vi "HFRR ADV v05.vi"() -> ()   [LabVIEW 2025] (continued)
    n981 = local read "Re-Initialise"() -> (w1097:bool)
    n982 = local read "Main Tab"() -> (w1093:T2)
    n983 = local read "service 3"() -> (w1094:bool)
    n984 = local read "OPEN 6"() -> (w1096:bool)
    n985 = local read "EDIT 2"() -> (w1099:bool)
    n986 = local read "RUN"() -> (w1111:bool)
    n987 = local read "RUN"() -> (w1109:bool)
    n988 = disable-structure shown="Disabled" {
      disable-tunnel: [w1126 _] -> w1091
      disable-tunnel: [w1125 _] -> w1089
      frame Disabled {
        n989 = local read "Temperature before test"() -> (w1119:dbl)
        n990 = local read "Temperature after test"() -> (w1132:dbl)
        n991 = case shown="True" "Save Results" {
          frame False {
          }
          frame True {
            w1148 = "\r"
            n992 = local write "Save Results"(FALSE ("OK Button 5")) -> ()
            n993 = local read "Temperature before test"() -> (w1186:dbl)
            n994 = local read "Temperature after test"() -> (w1188:dbl)
            n995 = local read "Humidity before test"() -> (w1185:dbl)
            n996 = local read "Humidity after test"() -> (w1187:dbl)
            n997 = local read "WS1.4"() -> (w1192:dbl)
            n998 = local read "AVP"() -> (w1190:dbl)
            n999 = Number To Fractional String(number=w1192, width (-)=i16 6, precision (6)=i16 1) -> (F-format string=w1152:string)  [unwired: 1 in]
            n1000 = local read "MWSD"() -> (w1189:dbl)
            n1001 = local read "String"() -> (w1181:string)
            n1002 = local read "FILE"() -> (w1184:string)
            n1003 = local read "HCF"() -> (w1191:dbl)
            n1004 = Number To Fractional String(number=w1185, width (-)=i16 6, precision (6)=i16 1) -> (F-format string=w1177:string)  [unwired: 1 in]
            n1005 = Number To Fractional String(number=w1186, width (-)=i16 6, precision (6)=i16 1) -> (F-format string=w1174:string)  [unwired: 1 in]
            n1006 = Number To Fractional String(number=w1187, width (-)=i16 6, precision (6)=i16 1) -> (F-format string=w1170:string)  [unwired: 1 in]
            n1007 = Number To Fractional String(number=w1188, width (-)=i16 6, precision (6)=i16 1) -> (F-format string=w1166:string)  [unwired: 1 in]
            n1008 = Number To Fractional String(number=w1190, width (-)=i16 6, precision (6)=i16 3) -> (F-format string=w1159:string)  [unwired: 1 in]
            n1009 = Concatenate Strings(w1181, w1184) -> (w1203:string)
            n1010 = Number To Fractional String(number=w1189, width (-)=i16 6, precision (6)=i16 1) -> (F-format string=w1163:string)  [unwired: 1 in]
            n1011 = Number To Fractional String(number=w1191, width (-)=i16 6, precision (6)=i16 2) -> (F-format string=w1157:string)  [unwired: 1 in]
            n1012 = Concatenate Strings("(" ("string"), w1152, ")Microns" ("string")) -> (w1151:string)
            n1013 = local read "REMARKS"() -> (w1183:string)
            "REMARKS 2" <- w1183
            n1014 = Concatenate Strings("(" ("string"), w1177, " ) % RH," ("string")) -> (w1178:string)
            n1015 = Concatenate Strings(w1157, ")" ("string")) -> (w1155:string)
            n1016 = Concatenate Strings("(" ("string"), w1174, ")  Deg C ," ("string")) -> (w1173:string)
            n1017 = Concatenate Strings("(" ("string"), w1170, " ) % RH," ("string")) -> (w1169:string)
            n1018 = Concatenate Strings("(" ("string"), w1166, ")  Deg C ," ("string")) -> (w1165:string)
            n1019 = Concatenate Strings("(" ("string"), w1163, ")  Microns," ("string")) -> (w1162:string)
            n1020 = Concatenate Strings("(" ("string"), w1159, ")  kPa," ("string")) -> (w1149:string)
            n1021 = Concatenate Strings(w1203, ".dwm" ("Substring")) -> (w1201:string)
            n1022 = String To Path(string=w1201) -> (path=w1200:path)
            n1023 = Concatenate Strings(w1183, w1148, " Humidity before test= " ("Substring"), w1178, w1148, " Temperature before test = " ("Substring"), w1173, w1148, " Humidity after test= " ("Substring"), w1169, w1148, "Temperature after test = " ("Substring"), w1165, w1148, "MSD = " ("Substring"), w1162, w1148, "  AVP = " ("Substring"), w1149, w1148, "  HCF                     =( " ("Substring"), w1155, w1148, " WS1.4                  = " ("Substring"), w1151, w1148) -> (w1147:string)
            "data" <- w1147
            n1024 = call <vilib>:"Write Characters To File.vi"("append to file? (new file:F)"=FALSE, "character string"=w1147, "file path (dialog if empty)"=w1200) -> ()  [unwired: 2 in, 1 out]
            n1025 = Match Pattern(string=w1147, regular expression="!") -> (after substring=→"export":string)  [unwired: 1 in, 3 out]
          }
        }
        n1026 = Add(x=231.864, y=w1119) -> (x+y=w1116:dbl)
        n1027 = Add(x=231.864, y=w1132) -> (x+y=w1129:dbl)
        n1028 = Divide(x=1705.984, y=w1116) -> (x/y=w1117:dbl)
        n1029 = Divide(x=1705.984, y=w1129) -> (x/y=w1130:dbl)
        n1030 = local read "Humidity before test"() -> (w1121:dbl)
        n1031 = local read "Humidity after test"() -> (w1134:dbl)
        n1032 = Subtract(x=8.017352 ("y"), y=w1117) -> (x-y=w1143:dbl)
        n1033 = Subtract(x=8.017352 ("y"), y=w1130) -> (x-y=w1137:dbl)
        n1034 = expression code="10**y"(w1143) -> (w1123:dbl)
        n1035 = expression code="10**y"(w1137) -> (w1136:dbl)
        n1036 = Multiply(x=w1121, y=w1123) -> (x*y=w1122:dbl)
        n1037 = Multiply(x=w1134, y=w1136) -> (x*y=w1135:dbl)
        n1038 = Divide(x=w1122, y=750.0) -> (x/y=w1138:dbl)
        n1039 = Divide(x=w1135, y=750.0) -> (x/y=w1139:dbl)
        n1040 = Add(x=w1138, y=w1139) -> (x+y=w1140:dbl)
        n1041 = Divide(x=w1140, y=2.0) -> (x/y=w1142:dbl)
        n1042 = local write "AVP"(w1142) -> ()
        n1043 = Subtract(x=1.4, y=w1142) -> (x-y=w1125:dbl)
        n1044 = local read "HCF"() -> (w1126:dbl)
      }
      frame Enabled {
      }
    }
    n1045 = case shown="True" "EDIT 3" {
      frame False {
      }
      frame True {
        n1046 = local write "EDIT 3"(FALSE ("EDIT 3")) -> ()
        n1047 = local write "Main Tab"(T2."About" ("Main Tab")) -> ()
      }
    }
    n1048 = case shown="True" w1097 {
      frame False {
      }
      frame True {
        n1049 = local write "Re-Initialise"(FALSE ("Re-Initialise")) -> ()
      }
    }
    n1050 = case shown="False" w1111 {
      frame False {
        n1051 = local read "stopT"() -> (w2092:bool)
        n1052 = case shown="True" w2092 {
          frame False {
          }
          frame True {
            w2093 = FALSE
            n1053 = local write "stopT"(w2093) -> ()
            n1054 = local write "st enable"(w2093) -> ()
          }
        }
      }
      frame True {
        "stopT" <- TRUE
      }
    }
    n1055 = case shown="True" w1109 {
      frame False {
      }
      frame True {
        n1056 = local read "Main Tab"() -> (w2090:T2)
        n1057 = case shown="\"Compare Files\"" w2090 {
          frame "Acquire", Default {
          }
          frame "Compare Files" {
            n1058 = local write "Main Tab"(T2."Acquire" ("Main Tab")) -> ()
          }
          frame "About" {
          }
        }
      }
    }
    n1059 = case shown="True" w1099 {
      frame False {
        n1060 = property on="Password 2" class="Str"("Visible"=FALSE) -> ()  [unwired: 2 in, 2 out]
        n1061 = local write "Password 2"("" ("Password")) -> ()
      }
      frame True {
        n1062 = property on="Password 2" class="Str"("Visible"=TRUE) -> ()  [unwired: 2 in, 2 out]
        n1063 = Equal?(x="Password 2", y="HFRR1234") -> (x = y?=w1232:bool)
        n1064 = case shown="True" w1232 {
          tunnel: "Password 2" -> [w1235 _]
          frame False {
            n1065 = String Length(string=w1235) -> (length=w1236:i32)
            n1066 = Greater Than 0?(x=w1236) -> (x > 0?=w1234:bool)
            n1067 = case shown="False" w1234 {
              frame False {
                n1068 = property on="Password 2" class="Str"("Caption.Text"="Password (Advance Setting)") -> ()  [unwired: 2 in, 2 out]
              }
              frame True {
                n1069 = property on="Password 2" class="Str"("Caption.Text"="Incorrect Password!") -> ()  [unwired: 2 in, 2 out]
              }
            }
          }
          frame True {
            n1070 = local write "EDIT 2"(FALSE ("EDIT 2")) -> ()
            n1071 = local write "Password 2"("" ("Password")) -> ()
            n1072 = local write "Main Tab"(T2."Advance" ("Main Tab")) -> ()
          }
        }
      }
    }
    n1073 = case shown="True" "Prog Uno" {
      frame False {
      }
      frame True {
        n1074 = stacked-sequence {
          frame #0 {
            n1075 = Delete(path (use dialog)=path "C:/LAB-IQ-NXT/UNOCOMPILE.bat" ("working directory")) -> ()  [unwired: 4 in, 3 out]
          }
          frame #1 {
            n1076 = local read "Com Port 1"() -> (w1696:refnum<visa-resource-name>)
            n1077 = Concatenate Strings("cmd.exe /c \"mode " ("command line"), w1696, ":1200,n,8,1\"\n" ("command line")) -> (w1701:string)
            n1078 = Concatenate Strings(w1701, "CD\\\nCD WinDucom\navrdude -C avrdude.conf -v -patmega328p -carduino -P" ("command line"), w1696, " -b115200 -D -Uflash:w:UNO_V20.hex:i\n" ("command line"), "\r") -> (w1703:string)
            "STR" <- w1703
            n1079 = call <vilib>:"Write Characters To File.vi"("append to file? (new file:F)"=FALSE, "character string"=w1703, "file path (dialog if empty)"=path "C:/LAB-IQ-NXT/UNOCOMPILE.bat" ("working directory")) -> ()  [unwired: 2 in, 1 out]
          }
          frame #2 {
            n1080 = disable-structure shown="Disabled" {
              frame Disabled {
                w1707 = "cmd.exe  /c \"C:\\LAB-IQ-NXT\\UNOCOMPILE.bat\"" ("string")
                n1081 = local write "Prog Uno"(FALSE ("run minimized? (F)")) -> ()
                n1082 = call <vilib>:"System Exec.vi"("expected output size  (4096)"=u32 65535, "run minimized? (F)"=FALSE, "wait until completion? (T)"=TRUE ("run minimized? (F)"), "working directory"=path "C:/LAB-IQ-NXT", "standard input"=w1707, "command line"=w1707) -> ("error out"=w1706:errorcluster, "standard output"=→"String 42":string)  [unwired: 2 in, 2 out]
                "error out 3" <- w1706
                n1083 = flat-sequence {
                  tunnel: w1706 -> [_]
                  frame #0 {
                  }
                }
              }
              frame Enabled {
              }
            }
          }
        }
      }
    }
    n1084 = case shown="\"CEC F-096-A-06\"" "TEST STANDARD" {
      tunnel: [2.0 ("Set Temp") 0.0 ("Set Temp") 2.0 ("Set Temp") 0.0 ("Set Temp")] -> w1100
      frame "ASTM D6079", Default {
        # "astm hide"
        n1085 = local write "NORMAL LOAD"(2.0 ("NORMAL LOAD")) -> ()
        n1086 = local write "Set Strk"(1.0 ("Set Strk")) -> ()
        n1087 = local write "Set Hz"(50.0 ("Hz")) -> ()
        n1088 = local write "Set Temp"(60.0 ("Set Temp")) -> ()
        n1089 = local write "Set Rh"(53.0 ("Set Rh")) -> ()
        n1090 = local write "test time"(75.0 ("test time")) -> ()
        "Test Standard" <- "ASTM D6079" ("Test Standard 2")
      }
      frame "ISO 12156" {
        n1091 = local write "Set Strk"(1.0 ("Set Strk")) -> ()
        n1092 = local write "NORMAL LOAD"(2.0 ("NORMAL LOAD")) -> ()
        n1093 = local write "Set Temp"(60.0 ("Set Temp")) -> ()
        n1094 = local write "test time"(75.0 ("test time")) -> ()
        n1095 = local write "Set Hz"(50.0 ("Hz")) -> ()
        n1096 = local write "Set Rh"(53.0 ("Set Rh")) -> ()
      }
      frame "CEC F-096-A-06" {
        n1097 = local write "Set Strk"(1.0 ("Set Strk")) -> ()
        n1098 = local write "NORMAL LOAD"(2.0 ("NORMAL LOAD")) -> ()
        n1099 = local write "Set Temp"(60.0 ("Set Temp")) -> ()
        n1100 = local write "test time"(75.0 ("test time")) -> ()
        n1101 = local write "Set Hz"(50.0 ("Hz")) -> ()
        n1102 = local write "Set Rh"(53.0 ("Set Rh")) -> ()
      }
      frame "Custom" {
      }
    }
    n1103 = case shown="True" "Prog Due" {
      frame False {
      }
      frame True {
        n1104 = stacked-sequence {
          frame #0 {
            n1105 = Delete(path (use dialog)=path "C:/LAB-IQ-NXT/DUECOMPILE.bat" ("working directory")) -> ()  [unwired: 4 in, 3 out]
          }
          frame #1 {
            n1106 = disable-structure shown="Disabled" {
              frame Disabled {
                n1107 = local read "visa due"() -> (w1678:string)
                n1108 = Concatenate Strings("cmd.exe /c \"mode " ("command line"), w1678, ":1200,n,8,1\"\n" ("command line")) -> (w1683:string)
                n1109 = Concatenate Strings(w1683, "CD\\\nCD WinDucom\nTIMEOUT 1\n bossac.exe -i -d --port=" ("command line"), w1678, " -U false -e -w -v -b DUE.bin -R\n" ("command line"), "\r") -> (w1685:string)
                "concatenated string 2" <- w1685
                n1110 = call <vilib>:"Write Characters To File.vi"("append to file? (new file:F)"=FALSE, "character string"=w1685, "file path (dialog if empty)"=path "C:/LAB-IQ-NXT/DUECOMPILE.bat" ("working directory")) -> ()  [unwired: 2 in, 1 out]
              }
              frame Enabled {
              }
            }
          }
          frame #2 {
            # "C:\\LAB-IQ-NXT\\DUECOMPILE.bat"
            n1111 = disable-structure shown="Disabled" {
              frame Disabled {
                w1690 = "cmd.exe  /c \"C:\\LAB-IQ-NXT\\DUECOMPILE.bat\"" ("string")
                n1112 = call <vilib>:"System Exec.vi"("expected output size  (4096)"=u32 65535, "run minimized? (F)"=FALSE, "wait until completion? (T)"=TRUE ("run minimized? (F)"), "working directory"=path "C:/LAB-IQ-NXT", "standard input"=w1690, "command line"=w1690) -> ("error out"=w1689:errorcluster, "standard output"=→"String 44":string)  [unwired: 2 in, 2 out]
                "error out 4" <- w1689
                n1113 = flat-sequence {
                  tunnel: w1689 -> [_]
                  frame #0 {
                  }
                }
              }
              frame Enabled {
              }
            }
            n1114 = local write "Prog Due"(FALSE ("Prog Due")) -> ()
          }
        }
      }
    }
    n1115 = Or(x=w1096, y=w1094) -> (x .or. y?=w1095:bool)
    n1116 = case shown="\"About\"" w1093 {
      tunnel: [T15."Acquire" ("Main Tab") T15."Compare Files" ("Main Tab") T15."About" ("Main Tab")] -> w1107
      frame "Acquire", Default {
      }
      frame "Compare Files" {
      }
      frame "About" {
      }
    }
    n1117 = Or(x=w1101, y="OPEN") -> (x .or. y?=w1102:bool)
    n1118 = case shown="True" w1102 {
      tunnel: w1101 -> [_ w1242]
      frame False {
      }
      frame True {
        n1119 = stacked-sequence {
          tunnel: w1242 -> [_ w1309 _ _]
          frame #0 {
            w1258 = "  " ("String 6")
            n1120 = local write "OPEN"(FALSE ("open")) -> ()
            n1121 = local read "string1 2"() -> (w1246:string)
            n1122 = local read "string1 3"() -> (w1245:string)
            n1123 = local read "string1 4"() -> (w1244:string)
            n1124 = property on="OPEN" class="Bool (strict)"("Visible"=FALSE) -> ()  [unwired: 2 in, 2 out]
            n1125 = local write "String 6"(w1258) -> ()
            n1126 = local write "String 7"(w1258) -> ()
            n1127 = local write "String 8"(w1258) -> ()
            n1128 = local write "String 12"(w1258) -> ()
            n1129 = local read "OK Button 16"() -> (w1243:bool)
            n1130 = String To Path(string=w1246) -> (path=w1254:path)
            n1131 = String To Path(string=w1245) -> (path=w1253:path)
            n1132 = String To Path(string=w1244) -> (path=w1252:path)
            n1133 = case shown="True" w1243 {
              tunnel: [w1259 w1260] -> w1247
              frame False {
                n1134 = local read "string1"() -> (w1259:string)
              }
              frame True {
                n1135 = local read "String Indicator 4"() -> (w1260:string)
              }
            }
            n1136 = Open/Create/Replace File "Open File"(file path (use dialog)=w1254) -> (refnum out=w1250:refnum<file>)  [unwired: 5 in, 2 out]
            n1137 = Open/Create/Replace File "Open File"(file path (use dialog)=w1253) -> (refnum out=w1249:refnum<file>)  [unwired: 5 in, 2 out]
            n1138 = Open/Create/Replace File "Open File"(file path (use dialog)=w1252) -> (refnum out=w1248:refnum<file>)  [unwired: 5 in, 2 out]
            n1139 = while {
              tunnel: w1250 -> [w1272]
              i -> [w1268]
              stop <- w1267 continue-if-true
              (unwired) TRUE ("line mode (F)")
              n1140 = Read from Text File "Read File"(file (use dialog)=w1272) -> (text=w1269:string)  [unwired: 3 in, 3 out]
              n1141 = local write "Numeric 11"(w1268) -> ()
              n1142 = String Length(string=w1269) -> (length=w1271:i32)
              n1143 = Greater?(x=w1271, y=1) -> (0:w1267:bool)
            }
            n1144 = while {
              tunnel: w1249 -> [w1278]
              i -> [w1274]
              stop <- w1273 continue-if-true
              (unwired) TRUE ("line mode (F)")
              n1145 = Read from Text File "Read File"(file (use dialog)=w1278) -> (text=w1275:string)  [unwired: 3 in, 3 out]
              n1146 = local write "Numeric 12"(w1274) -> ()
              n1147 = String Length(string=w1275) -> (length=w1277:i32)
              n1148 = Greater?(x=w1277, y=1) -> (0:w1273:bool)
            }
            n1149 = while {
              tunnel: w1248 -> [w1284]
              i -> [w1280]
              stop <- w1279 continue-if-true
              (unwired) TRUE ("line mode (F)")
              n1150 = Read from Text File "Read File"(file (use dialog)=w1284) -> (text=w1281:string)  [unwired: 3 in, 3 out]
              n1151 = local write "Numeric 13"(w1280) -> ()
              n1152 = String Length(string=w1281) -> (length=w1283:i32)
              n1153 = Greater?(x=w1283, y=1) -> (0:w1279:bool)
            }
            n1154 = String To Path(string=w1247) -> (path=w1255:path)
            n1155 = Open/Create/Replace File "Open File"(file path (use dialog)=w1255) -> (refnum out=w1251:refnum<file>)  [unwired: 5 in, 2 out]
            n1156 = while {
              tunnel: w1251 -> [w1266]
              i -> [w1262]
              stop <- w1261 continue-if-true
              (unwired) TRUE ("line mode (F)")
              n1157 = Read from Text File "Read File"(file (use dialog)=w1266) -> (text=w1263:string)  [unwired: 3 in, 3 out]
              n1158 = local write "Numeric 8"(w1262) -> ()
              n1159 = String Length(string=w1263) -> (length=w1265:i32)
              n1160 = Greater?(x=w1265, y=1) -> (0:w1261:bool)
            }
          }
          frame #1 {
            w1436 = FALSE ("ACTUAL   MERGE")
            # "Sample Temp"
            # "ECR"
            # "COF"
            # "Time\nCOF\nFF\nTemp"
            n1161 = case shown="True" w1309 {
              tunnel: [w1456 w1457] -> w1310
              frame False {
                n1162 = local read "string1"() -> (w1456:string)
              }
              frame True {
                n1163 = local read "String Indicator 4"() -> (w1457:string)
              }
            }
            n1164 = local read "string1 3"() -> (w1354:string)
            n1165 = String To Path(string=w1310) -> (path=w1441:path)
            n1166 = String To Path(string=w1354) -> (path=w1452:path)
            n1167 = local read "Numeric 12"() -> (w1438:i32)
            n1168 = local read "Numeric 8"() -> (w1440:i32)
            n1169 = local read "string1 2"() -> (w1355:string)
            n1170 = local read "string1 4"() -> (w1353:string)
            n1171 = Open/Create/Replace File "Open File"(file path (use dialog)=w1441) -> (refnum out=w1455:refnum<file>, error out=w1454:errorcluster)  [unwired: 5 in, 1 out]
            n1172 = Open/Create/Replace File "Open File"(file path (use dialog)=w1452) -> (refnum out=w1448:refnum<file>, error out=w1449:errorcluster)  [unwired: 5 in, 1 out]
            n1173 = for {
              N: w1440 -> [_]
              tunnel: w1455 -> [w1603]
              tunnel: w1454 -> [w1602]
              tunnel: [w1592] -> w1367 mode=indexing
              tunnel: [w1590] -> w1424 mode=indexing
              tunnel: [w1591] -> w1419 mode=indexing
              tunnel: w1436 -> [_]
              tunnel: [w1584] -> w1421 mode=indexing
              tunnel: [w1580] -> w1390 mode=indexing
              tunnel: [w1576] -> w1365 mode=indexing
              tunnel: [w1572] -> w1346 mode=indexing
              tunnel: [w1567] -> w1306 mode=indexing
              (unwired) TRUE ("line mode (F)")
              # "freq"
              # "Stroke"
              # "Time"
              # "CoF"
              # "Humidity"
              # "Temp"
              # "Air Temp"
              # "ECR"
              n1174 = Read from Text File "Read File"(file (use dialog)=w1603, error in=w1602) -> (text=w1568:string)  [unwired: 2 in, 3 out]
              n1175 = local write "String 6"(w1568) -> ()
              n1176 = String Subset(string=w1568, offset (0)=0, length (rest)=14 ("length (rest)")) -> (substring=w1596:string)
              n1177 = String Subset(string=w1568, offset (0)=35, length (rest)=9 ("length (rest)")) -> (substring=w1593:string)
              n1178 = String Subset(string=w1568, offset (0)=15, length (rest)=9 ("length (rest)")) -> (substring=w1599:string)
              n1179 = Fract/Exp String To Number(string=w1596) -> (number=w1592:dbl)  [unwired: 3 in, 1 out]
              n1180 = Fract/Exp String To Number(string=w1593) -> (number=w1591:dbl)  [unwired: 3 in, 1 out]
              n1181 = Fract/Exp String To Number(string=w1599) -> (number=w1590:dbl)  [unwired: 3 in, 1 out]
              n1182 = String Subset(string=w1568, offset (0)=85, length (rest)=9 ("length (rest)")) -> (substring=w1569:string)
              n1183 = String Subset(string=w1568, offset (0)=25, length (rest)=9 ("length (rest)")) -> (substring=w1575:string)
              n1184 = String Subset(string=w1568, offset (0)=55, length (rest)=9 ("length (rest)")) -> (substring=w1577:string)
              n1185 = String Subset(string=w1568, offset (0)=45, length (rest)=9 ("length (rest)")) -> (substring=w1583:string)
              n1186 = String Subset(string=w1568, offset (0)=65, length (rest)=9 ("length (rest)")) -> (substring=w1589:string)
              n1187 = Fract/Exp String To Number(string=w1575) -> (number=w1572:dbl)  [unwired: 3 in, 1 out]
              n1188 = Fract/Exp String To Number(string=w1569) -> (number=w1567:dbl)  [unwired: 3 in, 1 out]
              n1189 = Fract/Exp String To Number(string=w1577) -> (number=w1576:dbl)  [unwired: 3 in, 1 out]
              n1190 = Fract/Exp String To Number(string=w1583) -> (number=w1580:dbl)  [unwired: 3 in, 1 out]
              n1191 = Fract/Exp String To Number(string=w1589) -> (number=w1586:dbl)  [unwired: 3 in, 1 out]
              n1192 = Add(x=w1586, y=0.0) -> (x+y=w1584:dbl)
            }
            n1193 = for {
              N: w1438 -> [_]
              tunnel: w1449 -> [w1529]
              tunnel: w1448 -> [w1528]
              tunnel: [w1518] -> w1407 mode=indexing
              tunnel: [w1516] -> w1405 mode=indexing
              tunnel: [w1517] -> w1401 mode=indexing
              tunnel: w1436 -> [_]
              tunnel: [w1510] -> w1403 mode=indexing
              tunnel: [w1506] -> w1385 mode=indexing
              tunnel: [w1502] -> w1361 mode=indexing
              tunnel: [w1499] -> w1342 mode=indexing
              tunnel: [w1495] -> w1301 mode=indexing
              (unwired) 9 ("length (rest)")
              (unwired) 9 ("length (rest)")
              (unwired) TRUE ("line mode (F)")
              n1194 = Read from Text File "Read File"(file (use dialog)=w1528, error in=w1529) -> (text=w1496:string)  [unwired: 2 in, 3 out]
              n1195 = local write "String 8"(w1496) -> ()
              n1196 = String Subset(string=w1496, offset (0)=85) -> (substring=w1498:string)  [unwired: 1 in]
              n1197 = String Subset(string=w1496, offset (0)=35, length (rest)=9 ("length (rest)")) -> (substring=w1519:string)
              n1198 = String Subset(string=w1496, offset (0)=55, length (rest)=9 ("length (rest)")) -> (substring=w1504:string)
              n1199 = String Subset(string=w1496, offset (0)=25) -> (substring=w1500:string)  [unwired: 1 in]
              n1200 = String Subset(string=w1496, offset (0)=15, length (rest)=9 ("length (rest)")) -> (substring=w1525:string)
              n1201 = String Subset(string=w1496, offset (0)=0, length (rest)=14 ("length (rest)")) -> (substring=w1522:string)
              n1202 = String Subset(string=w1496, offset (0)=45, length (rest)=9 ("length (rest)")) -> (substring=w1509:string)
              n1203 = String Subset(string=w1496, offset (0)=65, length (rest)=9 ("length (rest)")) -> (substring=w1515:string)
              n1204 = Fract/Exp String To Number(string=w1498) -> (number=w1495:dbl)  [unwired: 3 in, 1 out]
              n1205 = Fract/Exp String To Number(string=w1519) -> (number=w1517:dbl)  [unwired: 3 in, 1 out]
              n1206 = Fract/Exp String To Number(string=w1504) -> (number=w1502:dbl)  [unwired: 3 in, 1 out]
              n1207 = Fract/Exp String To Number(string=w1500) -> (number=w1499:dbl)  [unwired: 3 in, 1 out]
              n1208 = Fract/Exp String To Number(string=w1525) -> (number=w1516:dbl)  [unwired: 3 in, 1 out]
              n1209 = Fract/Exp String To Number(string=w1522) -> (number=w1518:dbl)  [unwired: 3 in, 1 out]
              n1210 = Fract/Exp String To Number(string=w1509) -> (number=w1506:dbl)  [unwired: 3 in, 1 out]
              n1211 = Fract/Exp String To Number(string=w1515) -> (number=w1512:dbl)  [unwired: 3 in, 1 out]
              n1212 = Add(x=w1512, y=0.0) -> (x+y=w1510:dbl)
            }
            n1213 = String To Path(string=w1355) -> (path=w1453:path)
            n1214 = String To Path(string=w1353) -> (path=w1447:path)
            n1215 = local read "Numeric 11"() -> (w1437:i32)
            n1216 = local read "Numeric 13"() -> (w1439:i32)
            n1217 = Open/Create/Replace File "Open File"(file path (use dialog)=w1453) -> (refnum out=w1451:refnum<file>, error out=w1450:errorcluster)  [unwired: 5 in, 1 out]
            n1218 = Open/Create/Replace File "Open File"(file path (use dialog)=w1447) -> (refnum out=w1446:refnum<file>, error out=w1445:errorcluster)  [unwired: 5 in, 1 out]
            n1219 = for {
              N: w1437 -> [_]
              tunnel: w1451 -> [w1566]
              tunnel: w1450 -> [w1565]
              tunnel: [w1555] -> w1417 mode=indexing
              tunnel: [w1553] -> w1415 mode=indexing
              tunnel: [w1554] -> w1410 mode=indexing
              tunnel: w1436 -> [_]
              tunnel: [w1547] -> w1412 mode=indexing
              tunnel: [w1543] -> w1388 mode=indexing
              tunnel: [w1539] -> w1363 mode=indexing
              tunnel: [w1535] -> w1344 mode=indexing
              tunnel: [w1530] -> w1302 mode=indexing
              (unwired) TRUE ("line mode (F)")
              n1220 = Read from Text File "Read File"(file (use dialog)=w1566, error in=w1565) -> (text=w1531:string)  [unwired: 2 in, 3 out]
              n1221 = local write "String 7"(w1531) -> ()
              n1222 = String Subset(string=w1531, offset (0)=85, length (rest)=9 ("length (rest)")) -> (substring=w1534:string)
              n1223 = String Subset(string=w1531, offset (0)=35, length (rest)=9 ("length (rest)")) -> (substring=w1556:string)
              n1224 = String Subset(string=w1531, offset (0)=55, length (rest)=9 ("length (rest)")) -> (substring=w1542:string)
              n1225 = String Subset(string=w1531, offset (0)=25, length (rest)=9 ("length (rest)")) -> (substring=w1536:string)
              n1226 = String Subset(string=w1531, offset (0)=45, length (rest)=9 ("length (rest)")) -> (substring=w1544:string)
              n1227 = String Subset(string=w1531, offset (0)=0, length (rest)=14 ("length (rest)")) -> (substring=w1559:string)
              n1228 = String Subset(string=w1531, offset (0)=15, length (rest)=9 ("length (rest)")) -> (substring=w1562:string)
              n1229 = String Subset(string=w1531, offset (0)=65, length (rest)=9 ("length (rest)")) -> (substring=w1548:string)
              n1230 = Fract/Exp String To Number(string=w1534) -> (number=w1530:dbl)  [unwired: 3 in, 1 out]
              n1231 = Fract/Exp String To Number(string=w1556) -> (number=w1554:dbl)  [unwired: 3 in, 1 out]
              n1232 = Fract/Exp String To Number(string=w1542) -> (number=w1539:dbl)  [unwired: 3 in, 1 out]
              n1233 = Fract/Exp String To Number(string=w1536) -> (number=w1535:dbl)  [unwired: 3 in, 1 out]
              n1234 = Fract/Exp String To Number(string=w1544) -> (number=w1543:dbl)  [unwired: 3 in, 1 out]
              n1235 = Fract/Exp String To Number(string=w1559) -> (number=w1555:dbl)  [unwired: 3 in, 1 out]
              n1236 = Fract/Exp String To Number(string=w1562) -> (number=w1553:dbl)  [unwired: 3 in, 1 out]
              n1237 = Fract/Exp String To Number(string=w1548) -> (number=w1551:dbl)  [unwired: 3 in, 1 out]
              n1238 = Add(x=w1551, y=0.0) -> (x+y=w1547:dbl)
            }
            n1239 = for {
              N: w1439 -> [_]
              tunnel: w1446 -> [w1494]
              tunnel: w1445 -> [w1493]
              tunnel: [w1483] -> w1399 mode=indexing
              tunnel: [w1482] -> w1392 mode=indexing
              tunnel: w1436 -> [_]
              tunnel: [w1471] -> w1397 mode=indexing
              tunnel: [w1476] -> w1394 mode=indexing
              tunnel: [w1472] -> w1384 mode=indexing
              tunnel: [w1467] -> w1359 mode=indexing
              tunnel: [w1463] -> w1340 mode=indexing
              tunnel: [w1458] -> w1300 mode=indexing
              (unwired) 1.0 ("x")
              (unwired) TRUE ("line mode (F)")
              n1240 = Read from Text File "Read File"(file (use dialog)=w1494, error in=w1493) -> (text=w1459:string)  [unwired: 2 in, 3 out]
              n1241 = local write "String 12"(w1459) -> ()
              n1242 = String Subset(string=w1459, offset (0)=85, length (rest)=9 ("length (rest)")) -> (substring=w1461:string)
              n1243 = String Subset(string=w1459, offset (0)=35, length (rest)=9 ("length (rest)")) -> (substring=w1484:string)
              n1244 = String Subset(string=w1459, offset (0)=55, length (rest)=9 ("length (rest)")) -> (substring=w1469:string)
              n1245 = String Subset(string=w1459, offset (0)=25, length (rest)=9 ("length (rest)")) -> (substring=w1465:string)
              n1246 = String Subset(string=w1459, offset (0)=45, length (rest)=9 ("length (rest)")) -> (substring=w1474:string)
              n1247 = String Subset(string=w1459, offset (0)=15, length (rest)=9 ("length (rest)")) -> (substring=w1490:string)
              n1248 = String Subset(string=w1459, offset (0)=0, length (rest)=14 ("length (rest)")) -> (substring=w1487:string)
              n1249 = String Subset(string=w1459, offset (0)=65, length (rest)=9 ("length (rest)")) -> (substring=w1477:string)
              n1250 = Fract/Exp String To Number(string=w1461) -> (number=w1458:dbl)  [unwired: 3 in, 1 out]
              n1251 = Fract/Exp String To Number(string=w1484) -> (number=w1482:dbl)  [unwired: 3 in, 1 out]
              n1252 = Fract/Exp String To Number(string=w1469) -> (number=w1467:dbl)  [unwired: 3 in, 1 out]
              n1253 = Fract/Exp String To Number(string=w1465) -> (number=w1463:dbl)  [unwired: 3 in, 1 out]
              n1254 = Fract/Exp String To Number(string=w1474) -> (number=w1472:dbl)  [unwired: 3 in, 1 out]
              n1255 = Fract/Exp String To Number(string=w1490) -> (number=w1471:dbl)  [unwired: 3 in, 1 out]
              n1256 = Fract/Exp String To Number(string=w1487) -> (number=w1483:dbl)  [unwired: 3 in, 1 out]
              n1257 = Fract/Exp String To Number(string=w1477) -> (number=w1480:dbl)  [unwired: 3 in, 1 out]
              n1258 = Add(x=w1480, y=0.0) -> (x+y=w1476:dbl)
            }
            n1259 = Delete From Array(array=w1342, index=0) -> (array with subset deleted=w1315:dbl[])  [unwired: 1 in, 1 out]
            n1260 = Delete From Array(array=w1405, index=0) -> (array with subset deleted=w1378:dbl[])  [unwired: 1 in, 1 out]
            n1261 = Delete From Array(array=w1385, index=0) -> (array with subset deleted=w1373:dbl[])  [unwired: 1 in, 1 out]
            n1262 = Delete From Array(array=w1403, index=0) -> (array with subset deleted=w1404:dbl[])  [unwired: 1 in, 1 out]
            n1263 = call-poly <vilib>:"Mean.vi"("X"=w1315) -> ("mean"=→"КОФ2 4":dbl)  [unwired: 1 out]
            n1264 = call-poly <vilib>:"Mean.vi"("X"=w1378) -> ("mean"=→"КОФ3":dbl)  [unwired: 1 out]
            n1265 = call-poly <vilib>:"Mean.vi"("X"=w1373) -> ("mean"=→"CP3":dbl)  [unwired: 1 out]
            n1266 = Delete From Array(array=w1367, index=0) -> (array with subset deleted=w1294:dbl[])  [unwired: 1 in, 1 out]
            n1267 = Delete From Array(array=w1306, index=0) -> (array with subset deleted=w1293:dbl[])  [unwired: 1 in, 1 out]
            n1268 = Delete From Array(array=w1346, index=0) -> (array with subset deleted=w1317:dbl[])  [unwired: 1 in, 1 out]
            n1269 = Delete From Array(array=w1424, index=0) -> (array with subset deleted=w1379:dbl[])  [unwired: 1 in, 1 out]
            n1270 = Delete From Array(array=w1390, index=0) -> (array with subset deleted=w1375:dbl[])  [unwired: 1 in, 1 out]
            "array w/ subset deleted" <- w1375
            n1271 = Delete From Array(array=w1421, index=0) -> (array with subset deleted=w1422:dbl[])  [unwired: 1 in, 1 out]
            n1272 = call-poly <vilib>:"Mean.vi"("X"=w1317) -> ("mean"=→"КОФ2 2":dbl)  [unwired: 1 out]
            n1273 = call-poly <vilib>:"Mean.vi"("X"=w1379) -> ("mean"=→"КОФ1":dbl)  [unwired: 1 out]
            n1274 = Bundle "Bundle"(w1294, w1293) -> (w1299:cluster{dbl[], dbl[]})  [unwired: 1 in]
            n1275 = Bundle "Bundle"(w1294, w1422) -> (w1286:cluster{dbl[], dbl[]})  [unwired: 1 in]
            n1276 = Delete From Array(array=w1301, index=0) -> (array with subset deleted=w1289:dbl[])  [unwired: 1 in, 1 out]
            n1277 = Delete From Array(array=w1302, index=0) -> (array with subset deleted=w1291:dbl[])  [unwired: 1 in, 1 out]
            n1278 = Delete From Array(array=w1412, index=0) -> (array with subset deleted=w1413:dbl[])  [unwired: 1 in, 1 out]
            n1279 = Delete From Array(array=w1300, index=0) -> (array with subset deleted=w1287:dbl[])  [unwired: 1 in, 1 out]
            n1280 = Delete From Array(array=w1394, index=0) -> (array with subset deleted=w1395:dbl[])  [unwired: 1 in, 1 out]
            n1281 = Delete From Array(array=w1419, index=0) -> (array with subset deleted=w1325:dbl[])  [unwired: 1 in, 1 out]
            n1282 = Delete From Array(array=w1365, index=0) -> (array with subset deleted=w1321:dbl[])  [unwired: 1 in, 1 out]
            n1283 = Delete From Array(array=w1401, index=0) -> (array with subset deleted=w1323:dbl[])  [unwired: 1 in, 1 out]
            n1284 = Delete From Array(array=w1361, index=0) -> (array with subset deleted=w1319:dbl[])  [unwired: 1 in, 1 out]
            n1285 = Delete From Array(array=w1410, index=0) -> (array with subset deleted=w1324:dbl[])  [unwired: 1 in, 1 out]
            n1286 = Delete From Array(array=w1363, index=0) -> (array with subset deleted=w1320:dbl[])  [unwired: 1 in, 1 out]
            n1287 = Delete From Array(array=w1344, index=0) -> (array with subset deleted=w1316:dbl[])  [unwired: 1 in, 1 out]
            n1288 = Delete From Array(array=w1388, index=0) -> (array with subset deleted=w1374:dbl[])  [unwired: 1 in, 1 out]
            n1289 = Delete From Array(array=w1415, index=0) -> (array with subset deleted=w1376:dbl[])  [unwired: 1 in, 1 out]
            n1290 = Delete From Array(array=w1392, index=0) -> (array with subset deleted=w1322:dbl[])  [unwired: 1 in, 1 out]
            n1291 = Delete From Array(array=w1359, index=0) -> (array with subset deleted=w1318:dbl[])  [unwired: 1 in, 1 out]
            n1292 = Delete From Array(array=w1340, index=0) -> (array with subset deleted=w1314:dbl[])  [unwired: 1 in, 1 out]
            n1293 = Delete From Array(array=w1384, index=0) -> (array with subset deleted=w1372:dbl[])  [unwired: 1 in, 1 out]
            n1294 = Delete From Array(array=w1397, index=0) -> (array with subset deleted=w1377:dbl[])  [unwired: 1 in, 1 out]
            n1295 = Delete From Array(array=w1407, index=0) -> (array with subset deleted=w1290:dbl[])  [unwired: 1 in, 1 out]
            n1296 = Delete From Array(array=w1417, index=0) -> (array with subset deleted=w1292:dbl[])  [unwired: 1 in, 1 out]
            n1297 = Delete From Array(array=w1399, index=0) -> (array with subset deleted=w1288:dbl[])  [unwired: 1 in, 1 out]
            n1298 = Bundle "Bundle"(w1294, w1325) -> (w1312:cluster{dbl[], dbl[]})  [unwired: 1 in]
            n1299 = Bundle "Bundle"(w1294, w1379) -> (w1313:cluster{dbl[], dbl[]})  [unwired: 1 in]
            n1300 = Bundle "Bundle"(w1325, w1321) -> (w1327:cluster{dbl[], dbl[]})  [unwired: 1 in]
            n1301 = Bundle "Bundle"(w1290, w1289) -> (w1297:cluster{dbl[], dbl[]})  [unwired: 1 in]
            n1302 = Bundle "Bundle"(w1323, w1319) -> (w1329:cluster{dbl[], dbl[]})  [unwired: 1 in]
            n1303 = Bundle "Bundle"(w1290, w1323) -> (w1433:cluster{dbl[], dbl[]})  [unwired: 1 in]
            n1304 = Bundle "Bundle"(w1290, w1319) -> (w1357:cluster{dbl[], dbl[]})  [unwired: 1 in]
            n1305 = Bundle "Bundle"(w1290, w1378) -> (w1443:cluster{dbl[], dbl[]})  [unwired: 1 in]
            n1306 = Bundle "Bundle"(w1290, w1373) -> (w1381:cluster{dbl[], dbl[]})  [unwired: 1 in]
            n1307 = Bundle "Bundle"(w1290, w1404) -> (w1428:cluster{dbl[], dbl[]})  [unwired: 1 in]
            n1308 = Bundle "Bundle"(w1324, w1320) -> (w1328:cluster{dbl[], dbl[]})  [unwired: 1 in]
            n1309 = Bundle "Bundle"(w1292, w1291) -> (w1298:cluster{dbl[], dbl[]})  [unwired: 1 in]
            n1310 = Bundle "Bundle"(w1292, w1324) -> (w1435:cluster{dbl[], dbl[]})  [unwired: 1 in]
            n1311 = Bundle "Bundle"(w1292, w1320) -> (w1358:cluster{dbl[], dbl[]})  [unwired: 1 in]
            n1312 = Bundle "Bundle"(w1292, w1374) -> (w1382:cluster{dbl[], dbl[]})  [unwired: 1 in]
            n1313 = Bundle "Bundle"(w1292, w1376) -> (w1444:cluster{dbl[], dbl[]})  [unwired: 1 in]
            n1314 = Bundle "Bundle"(w1292, w1413) -> (w1426:cluster{dbl[], dbl[]})  [unwired: 1 in]
            n1315 = Bundle "Bundle"(w1322, w1318) -> (w1330:cluster{dbl[], dbl[]})  [unwired: 1 in]
            n1316 = Bundle "Bundle"(w1288, w1287) -> (w1296:cluster{dbl[], dbl[]})  [unwired: 1 in]
            n1317 = Bundle "Bundle"(w1288, w1322) -> (w1434:cluster{dbl[], dbl[]})  [unwired: 1 in]
            n1318 = Bundle "Bundle"(w1288, w1318) -> (w1356:cluster{dbl[], dbl[]})  [unwired: 1 in]
            n1319 = Bundle "Bundle"(w1288, w1372) -> (w1380:cluster{dbl[], dbl[]})  [unwired: 1 in]
            n1320 = Bundle "Bundle"(w1288, w1377) -> (w1442:cluster{dbl[], dbl[]})  [unwired: 1 in]
            n1321 = Bundle "Bundle"(w1288, w1395) -> (w1427:cluster{dbl[], dbl[]})  [unwired: 1 in]
            n1322 = call-poly <vilib>:"Mean.vi"("X"=w1375) -> ("mean"=→"CP1":dbl)  [unwired: 1 out]
            n1323 = call-poly <vilib>:"Mean.vi"("X"=w1316) -> ("mean"=→"КОФ2 3":dbl)  [unwired: 1 out]
            n1324 = call-poly <vilib>:"Mean.vi"("X"=w1374) -> ("mean"=→"CP2":dbl)  [unwired: 1 out]
            n1325 = call-poly <vilib>:"Mean.vi"("X"=w1376) -> ("mean"=→"КОФ2":dbl)  [unwired: 1 out]
            n1326 = call-poly <vilib>:"Mean.vi"("X"=w1314) -> ("mean"=→"КОФ2 5":dbl)  [unwired: 1 out]
            n1327 = call-poly <vilib>:"Mean.vi"("X"=w1372) -> ("mean"=→"CP4":dbl)  [unwired: 1 out]
            n1328 = call-poly <vilib>:"Mean.vi"("X"=w1377) -> ("mean"=→"КОФ4":dbl)  [unwired: 1 out]
            n1329 = Bundle "Bundle"(w1294, w1321) -> (w1285:cluster{dbl[], dbl[]})  [unwired: 1 in]
            n1330 = Bundle "Bundle"(w1294, w1375) -> (w1308:cluster{dbl[], dbl[]})  [unwired: 1 in]
            n1331 = Build Array "Build Array"(w1285, w1308) -> (w1311:cluster{dbl[], dbl[]}[])
            "XY Graph 17" <- w1311
            n1332 = Build Array "Build Array"(w1299, w1298, w1297, w1296) -> (→"Frequency":cluster{dbl[], dbl[]}[])
            n1333 = Build Array "Build Array"(w1327, w1328, w1329, w1330) -> (→"Air Temp vs Rh":cluster{dbl[], dbl[]}[])
            n1334 = Build Array "Build Array"(w1312, w1435, w1433, w1434) -> (→"Air Temperature":cluster{dbl[], dbl[]}[])
            n1335 = Build Array "Build Array"(w1285, w1358, w1357, w1356) -> (→"Humidity":cluster{dbl[], dbl[]}[])
            n1336 = Build Array "Build Array"(w1313, w1444, w1443, w1442) -> (→"Coefficient Of Friction":cluster{dbl[], dbl[]}[])
            n1337 = Build Array "Build Array"(w1308, w1382, w1381, w1380) -> (→"Sample Temperature":cluster{dbl[], dbl[]}[])
            n1338 = Build Array "Build Array"(w1286, w1426, w1428, w1427) -> (→"XY Graph 13":cluster{dbl[], dbl[]}[])
            n1339 = Bundle "Bundle"(w1294, w1317) -> (w1339:cluster{dbl[], dbl[]})  [unwired: 1 in]
            n1340 = Bundle "Bundle"(w1290, w1315) -> (w1337:cluster{dbl[], dbl[]})  [unwired: 1 in]
            n1341 = Bundle "Bundle"(w1292, w1316) -> (w1338:cluster{dbl[], dbl[]})  [unwired: 1 in]
            n1342 = Bundle "Bundle"(w1288, w1314) -> (w1336:cluster{dbl[], dbl[]})  [unwired: 1 in]
            n1343 = Build Array "Build Array"(w1339, w1338, w1337, w1336) -> (→"Stroke":cluster{dbl[], dbl[]}[])
            n1344 = local write "XY Graph 16"(w1311) -> ()
          }
          frame #2 {
          }
          frame #3 {
            n1345 = local write "Numeric 8"(0 ("Numeric 8")) -> ()
            n1346 = local write "Numeric 11"(0 ("Numeric 11")) -> ()
            n1347 = local write "Numeric 12"(0 ("Numeric 12")) -> ()
            n1348 = local write "Numeric 13"(0 ("Numeric 13")) -> ()
            n1349 = property on="OPEN" class="Bool (strict)"("Visible"=TRUE) -> ()  [unwired: 2 in, 2 out]
            n1350 = local read "String Control 2"() -> (w1611:string)
            n1351 = local read "String Control 4"() -> (w1610:string)
            n1352 = local read "String Control 6"() -> (w1609:string)
            n1353 = local read "String Control 8"() -> (w1608:string)
            n1354 = Match Pattern(string=w1611, regular expression="Samples / cycle :- ") -> (after substring=w1625:string)  [unwired: 1 in, 3 out]
            n1355 = Match Pattern(string=w1611, regular expression="Frequency :- ") -> (after substring=w1644:string)  [unwired: 1 in, 3 out]
            n1356 = Match Pattern(string=w1610, regular expression="Samples / cycle :- ") -> (after substring=w1621:string)  [unwired: 1 in, 3 out]
            n1357 = Match Pattern(string=w1610, regular expression="Frequency :- ") -> (after substring=w1639:string)  [unwired: 1 in, 3 out]
            n1358 = Match Pattern(string=w1609, regular expression="Samples / cycle :- ") -> (after substring=w1617:string)  [unwired: 1 in, 3 out]
            n1359 = Match Pattern(string=w1609, regular expression="Frequency :- ") -> (after substring=w1634:string)  [unwired: 1 in, 3 out]
            n1360 = Match Pattern(string=w1608, regular expression="Samples / cycle :- ") -> (after substring=w1613:string)  [unwired: 1 in, 3 out]
            n1361 = Match Pattern(string=w1608, regular expression="Frequency :- ") -> (after substring=w1629:string)  [unwired: 1 in, 3 out]
            n1362 = String Subset(string=w1625, length (rest)=6 ("length (rest)")) -> (substring=w1627:string)  [unwired: 1 in]
            n1363 = String Subset(string=w1644, length (rest)=9 ("length (rest)")) -> (substring=w1646:string)  [unwired: 1 in]
            n1364 = String Subset(string=w1621, length (rest)=6 ("length (rest)")) -> (substring=w1623:string)  [unwired: 1 in]
            n1365 = String Subset(string=w1639, length (rest)=9 ("length (rest)")) -> (substring=w1641:string)  [unwired: 1 in]
            n1366 = String Subset(string=w1617, length (rest)=6 ("length (rest)")) -> (substring=w1619:string)  [unwired: 1 in]
            n1367 = String Subset(string=w1634, length (rest)=9 ("length (rest)")) -> (substring=w1636:string)  [unwired: 1 in]
            n1368 = String Subset(string=w1613, length (rest)=6 ("length (rest)")) -> (substring=w1615:string)  [unwired: 1 in]
            n1369 = String Subset(string=w1629, length (rest)=9 ("length (rest)")) -> (substring=w1631:string)  [unwired: 1 in]
            n1370 = Fract/Exp String To Number(string=w1627) -> (number=w1607:dbl)  [unwired: 3 in, 1 out]
            n1371 = Fract/Exp String To Number(string=w1646) -> (number=w1647:dbl)  [unwired: 3 in, 1 out]
            n1372 = Fract/Exp String To Number(string=w1623) -> (number=w1606:dbl)  [unwired: 3 in, 1 out]
            n1373 = Fract/Exp String To Number(string=w1641) -> (number=w1642:dbl)  [unwired: 3 in, 1 out]
            n1374 = Fract/Exp String To Number(string=w1619) -> (number=w1605:dbl)  [unwired: 3 in, 1 out]
            n1375 = Fract/Exp String To Number(string=w1636) -> (number=w1637:dbl)  [unwired: 3 in, 1 out]
            n1376 = Fract/Exp String To Number(string=w1615) -> (number=w1604:dbl)  [unwired: 3 in, 1 out]
            n1377 = Fract/Exp String To Number(string=w1631) -> (number=w1632:dbl)  [unwired: 3 in, 1 out]
            n1378 = local write "sample1"(w1607) -> ()
            n1379 = local write "freq1"(w1647) -> ()
            n1380 = local write "sample2"(w1606) -> ()
            n1381 = local write "freq2"(w1642) -> ()
            n1382 = local write "sample3"(w1605) -> ()
            n1383 = local write "freq3"(w1637) -> ()
            n1384 = local write "sample4"(w1604) -> ()
            n1385 = local write "freq 4"(w1632) -> ()
          }
        }
      }
    }
    n1386 = case shown="True" w1095 {
      selector: w1095 -> [_ w1224]
      frame False {
      }
      frame True {
        n1387 = Not(x=w1224) -> (.not. x?=w1220:bool)
        n1388 = local write "service 3"(w1220) -> ()
        n1389 = local write "OPEN 6"(w1220) -> ()
        n1390 = call <vilib>:"System Exec.vi"("wait until completion? (T)"=TRUE, "command line"="C:\\LAB-IQ-NXT\\Scar View.exe") -> ("error out"=→"error out 5":errorcluster)  [unwired: 6 in, 3 out]
      }
    }
    n1391 = case shown="\"About\"" w1107 {
      frame "Acquire", Default {
        w2123 = 0.2 ("y")
        w2128 = 1.0 ("y")
        w2129 = 0.8 ("y")
        # "Elapsed time\ncof\nstroke\nAir temp\nTemp\nHumidity"
        n1392 = disable-structure shown="Disabled" {
          frame Disabled {
            n1393 = local read "Flag"() -> (w2146:dbl)
            n1394 = local read "RUN"() -> (w2143:bool)
            n1395 = Not(x=w2143) -> (.not. x?=w2142:bool)
            n1396 = Equal?(x=w2146, y=10.0) -> (x = y?=w2144:bool)
            n1397 = And(x=w2144, y=w2142) -> (x .and. y?=w2141:bool)
            n1398 = case shown="True" w2141 {
              frame False {
              }
              frame True {
                w2147 = FALSE ("Heater Button")
                n1399 = local write "Humidity"(w2147) -> ()
                n1400 = local write "Heater Button"(w2147) -> ()
              }
            }
          }
          frame Enabled {
          }
        }
        n1401 = disable-structure shown="Disabled" {
          frame Disabled {
            n1402 = case shown="True" {
              selector: _ -> [_ _]
              frame False {
              }
              frame True {
                w2238 = TRUE ("Heater")
                n1403 = local write "Humidity"(w2238) -> ()
                n1404 = local write "Heater Button"(w2238) -> ()
                n1405 = local read "TEST STANDARD"() -> (w2241:T3)
                n1406 = local read "TEST STANDARD"() -> (w2236:T3)
                n1407 = Equal?(x=w2241, y=enum16{"ASTM D6079", "ISO 12156", "Custom"}."ISO 12156" ("Test Standard")) -> (x = y?=w2239:bool)
                n1408 = Equal?(x=w2236, y=enum16{"ASTM D6079", "ISO 12156", "Custom"}."ASTM D6079" ("Test Standard")) -> (x = y?=w2235:bool)
                n1409 = case shown="True" w2239 {
                  frame False {
                  }
                  frame True {
                    n1410 = local write "Heater"(TRUE ("Heater")) -> ()
                    n1411 = local write "airtempflg"(FALSE ("airtempflg")) -> ()
                  }
                }
                n1412 = case shown="True" w2235 {
                  frame False {
                  }
                  frame True {
                    n1413 = local write "Heater"(FALSE ("Heater")) -> ()
                    n1414 = local write "airtempflg"(TRUE ("airtempflg")) -> ()
                  }
                }
              }
            }
          }
          frame Enabled {
          }
        }
        n1415 = stacked-sequence {
          frame #0 {
            n1416 = case shown="True" "RST FF" {
              frame False {
              }
              frame True {
                w2304 = 0.0 ("X Scale.Range:Maximum")
                n1417 = property on="Frictional Force ( N )" class="WFChart (strict)"("XScale.Maximum"=600.0 ("X Scale.Range:Maximum"), "XScale.Minimum"=w2304, "YScale.Maximum"=10.0 ("Y Scale.Range:Maximum"), "YScale.Minimum"=w2304) -> ()  [unwired: 2 in, 2 out]
              }
            }
          }
          frame #1 {
            n1418 = case shown="True" "RST TEMP" {
              frame False {
              }
              frame True {
                n1419 = property on="Temperature ( Deg C )" class="WFChart (strict)"("XScale.Minimum"=0.0 ("X Scale.Range:Minimum"), "XScale.Maximum"=600.0 ("X Scale.Range:Maximum"), "YScale.Minimum"=0.0 ("Y Scale.Range:Minimum"), "YScale.Maximum"=100.0 ("Y Scale.Range:Maximum")) -> ()  [unwired: 2 in, 2 out]
              }
            }
          }
          frame #2 {
            n1420 = case shown="True" "RSTCOF" {
              frame False {
              }
              frame True {
                n1421 = property on="Coefficient of Friction" class="WFChart (strict)"("XScale.Minimum"=0.0 ("X Scale.Range:Minimum"), "XScale.Maximum"=600.0 ("X Scale.Range:Maximum"), "YScale.Maximum"=1.0 ("X Scale.Range:Minimum"), "YScale.Minimum"=0.0 ("X Scale.Range:Minimum")) -> ()  [unwired: 2 in, 2 out]
              }
            }
          }
          frame #3 {
            n1422 = case shown="True" "RSTCOF 2" {
              frame False {
              }
              frame True {
                (unwired) 100.0 ("Y Scale.Range:Maximum")
                (unwired) 0.0 ("Y Scale.Range:Minimum")
                (unwired) 600.0 ("X Scale.Range:Maximum")
                (unwired) 0.0 ("X Scale.Range:Minimum")
              }
            }
          }
          frame #4 {
            n1423 = case shown="True" "RSTCOF 3" {
              frame False {
              }
              frame True {
                n1424 = property on="Electrical Contact Resistance ( % )" class="WFChart (strict)"("XScale.Minimum"=0.0 ("X Scale.Range:Minimum"), "XScale.Maximum"=600.0 ("X Scale.Range:Maximum"), "YScale.Minimum"=0.0 ("Y Scale.Range:Minimum"), "YScale.Maximum"=100.0 ("Y Scale.Range:Maximum")) -> ()  [unwired: 2 in, 2 out]
              }
            }
          }
        }
        n1425 = disable-structure shown="Disabled" {
          frame Disabled {
            n1426 = case shown="False" {
              selector: _ -> [_ _]
              frame False {
              }
              frame True {
                n1427 = local read "zflag 2"() -> (w2205:dbl)
                n1428 = local read "yflag"() -> (w2207:dbl)
                n1429 = Equal?(x=w2207, y=2.0 ("tflag")) -> (x = y?=w2209:bool)
                n1430 = Equal?(x=w2205, y=3.0 ("tflag")) -> (x = y?=w2208:bool)
                n1431 = And(x=w2209, y=w2208) -> (x .and. y?=w2203:bool)
                n1432 = case shown="True" w2203 {
                  frame False {
                  }
                  frame True {
                    w2234 = 0.0 ("zflag")
                    n1433 = local write "zflag"(w2234) -> ()
                    n1434 = local write "zflag 2"(w2234) -> ()
                    n1435 = Delete(path (use dialog)=path "C:/LAB-IQ-NXT/WO 2449 TT.sig" ("file path (dialog if empty)")) -> (deleted path=w2233:path)  [unwired: 4 in, 2 out]
                    n1436 = Delete(path (use dialog)=path "C:/LAB-IQ-NXT/WO 2449 TRH.sig" ("file path (dialog if empty)")) -> (deleted path=w2228:path)  [unwired: 4 in, 2 out]
                    n1437 = local read "SEN.RUN HRS"() -> (w2220:dbl)
                    n1438 = local read "SENSOR TIME"() -> (w2218:dbl)
                    n1439 = call <vilib>:"compatOverwrite.vi"("overwrite (F)"=TRUE) -> ("overwrite?"=w2210:T18)
                    n1440 = call <vilib>:"compatOverwrite.vi"("overwrite (F)"=TRUE) -> ("overwrite?"=w2214:T18)
                    n1441 = local read "Total No. of Tests"() -> (w2221:dbl)
                    n1442 = Add(x=w2218, y=w2220) -> (x+y=w2219:dbl)
                    "SEN.RUN HRS" <- w2219
                    n1443 = Open/Create/Replace File(file path (use dialog)=w2233, operation (0:open)=w2210) -> (refnum out=w2211:refnum<file>, error out=w2212:errorcluster)  [unwired: 4 in, 1 out]
                    n1444 = Open/Create/Replace File(file path (use dialog)=w2228, operation (0:open)=w2214) -> (refnum out=w2215:refnum<file>, error out=w2216:errorcluster)  [unwired: 4 in, 1 out]
                    n1445 = Deny Access(4:w2212, 6:T16."deny none" ("deny mode (2)"), 7:w2211) -> (3:w2232:refnum<file>)  [unwired: 1 out]
                    n1446 = Deny Access(4:w2216, 6:T16."deny none" ("deny mode (2)"), 7:w2215) -> (3:w2224:refnum<file>)  [unwired: 1 out]
                    n1447 = Number To Decimal String(number=w2221) -> (decimal integer string=w2229:string)  [unwired: 1 in]
                    n1448 = Number To Decimal String(number=w2219) -> (decimal integer string=w2225:string)  [unwired: 1 in]
                    n1449 = Write to Binary File(file (use dialog)=w2232, data=w2229, 5:FALSE ("prepend array or string size? (T)")) -> ()  [unwired: 3 in, 3 out]
                    n1450 = Write to Binary File(file (use dialog)=w2224, data=w2225, 5:FALSE ("prepend array or string size? (T)")) -> ()  [unwired: 3 in, 3 out]
                  }
                }
              }
            }
          }
          frame Enabled {
          }
        }
        n1451 = local read "RUN"() -> (w2132:bool)
        n1452 = local read "run replace"() -> (w2136:bool)
        n1453 = local read "run replace"() -> (w2135:bool)
        n1454 = case shown="True" w2132 {
          frame False {
            n1455 = local write "run replace"(FALSE ("run replace")) -> ()
          }
          frame True {
            "run replace" <- TRUE ("run replace")
          }
        }
        n1456 = local read "RUN"() -> (w2140:bool)
        n1457 = local read "Set Temp"() -> (w2102:dbl)
        n1458 = local read "SetTemp"() -> (w2104:dbl)
        n1459 = case shown="False" w2140 {
          tunnel: [FALSE ("TEST RUNNING") TRUE ("TEST RUNNING")] -> w2139
          frame False {
            w2323 = 0.0 ("Flag")
            n1460 = local write "Elapsed time"(0.0 ("elapsedtime")) -> ()
            n1461 = local write "Time Remaining"(w2323) -> ()
            n1462 = local write "Flag"(w2323) -> ()
          }
          frame True {
            n1463 = local write "Flag"(10.0 ("Flag")) -> ()
          }
        }
        n1464 = case shown="False" w2136 {
          frame False {
            n1465 = local read "zflag"() -> (→"zflag 2":dbl)
            n1466 = local write "yflag"(2.0 ("tflag")) -> ()
            n1467 = local write "FLAG 4"(0.0 ("FLAG")) -> ()
          }
          frame True {
